vi "MGCC_StaEst_zeroinjec.vi"(0 "A":dbl[][](array[numeric])) -> (1 "Node_ZeroInjec":i32[][](array[numeric]), 2 "Num_ZeroInjec":i32)   [LabVIEW 2016]
uses:
  <vilib>/imath/engines/lvmath2/RunTimeEngine/IndexRead/NIMS M($,S).vi
  <instcachedir>/0/NIMS M($,S)_3E5749BBB62E49528D4765A77F1F6D98.lvgen/NIMS M($,S)_3E5749BBB62E49528D4765A77F1F6D98_000.vi
  <vilib>/imath/engines/lvmath2/RunTimeEngine/BuiltInFunctions/findnz/NIMS_[1o]_findnz(GColV).vi
  <instcachedir>/0/NIMS_[1o]_findnz(GColV)_8556557C9365446B906472366DD9B2D8.lvgen/NIMS_[1o]_findnz(GColV)_8556557C9365446B906472366DD9B2D8_000.vi
  <vilib>/imathl/engines/lvmath/Functions/Error Handling/Create Error.vi
  <vilib>/imath/engines/lvmath2/RunTimeEngine/BuiltInFunctions/size/NIMS_I32=size(GCol,I32).vi
  <instcachedir>/0/NIMS_I32=size(GCol,I32)_3BEAC9C04C22472CB193ADA08E7FE41C.lvgen/NIMS_I32=size(GCol,I32)_3BEAC9C04C22472CB193ADA08E7FE41C_000.vi
  <vilib>/imath/engines/lvmath2/RunTimeEngine/BuiltInFunctions/ones/NIMS_V=ones(I32,I32).vi
  <vilib>/imath/engines/lvmath2/RunTimeEngine/RowToken/NIMS_RowToken_CV_CV.vi
  <instcachedir>/0/NIMS_RowToken_CV_CV_5546A0B1CA2C4E49826F811B9C073FB0.lvgen/NIMS_RowToken_CV_CV_5546A0B1CA2C4E49826F811B9C073FB0_002.vi
  <vilib>/imath/engines/lvmath2/RunTimeEngine/ErrorHandling/NIMS_Create Error From Enums.vi
  <vilib>/imath/engines/lvmath2/RunTimeEngine/NodeEndStatement/NIMS_NodeEndStatement_Output.vi
  <instcachedir>/0/NIMS_NodeEndStatement_Output_53EC0D466D134D7ABD903AC30B43404B.lvgen/NIMS_NodeEndStatement_Output_53EC0D466D134D7ABD903AC30B43404B_011.vi
  <instcachedir>/0/NIMS_NodeEndStatement_Output_53EC0D466D134D7ABD903AC30B43404B.lvgen/NIMS_NodeEndStatement_Output_53EC0D466D134D7ABD903AC30B43404B_013.vi
  <vilib>/imath/engines/lvmath2/RunTimeEngine/ErrorHandling/NIMS_Finalize Error.vi
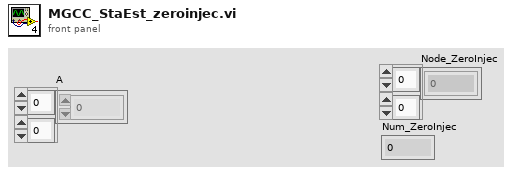
[diagram p1: front panel]
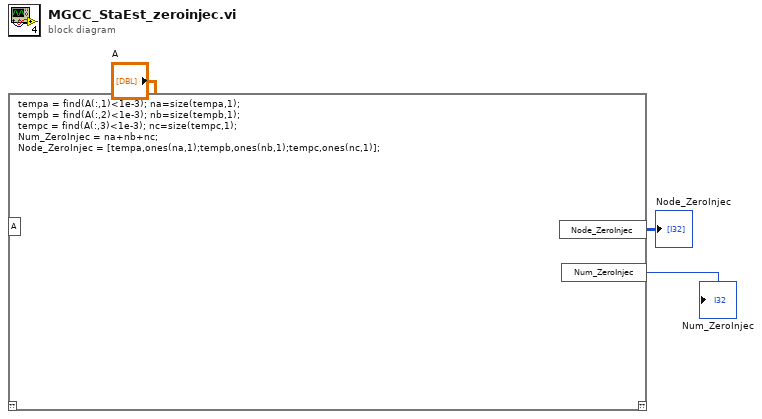
[diagram p0: block diagram]
diagram:
  n1 = mathscript code="tempa = find(A(:,1)<1e-3); na=size(tempa,1);\ntempb = find(A(:,2)<1e-3); nb=size(tempb,1);\ntempc = find(A(:,3)<1e-3); nc=size(tempc,1);\nNum_ZeroInjec = na+nb+nc;\nNode_ZeroInjec = [tempa,ones(na,1);tempb,ones(nb,1);tempc,ones(nc,1)];"("A"="A") -> ("Node_ZeroInjec"=→"Node_ZeroInjec":i32[][], "Num_ZeroInjec"=→"Num_ZeroInjec":i32)  [unwired: 1 in, 1 out]
